vi "isUpperLevelClosed.vi"(8 "error in (no error)":errorcluster, 9 "open nodes":refnum<class "xmlNode.lvclass">[](array[class]), 10 "open names":string[](array[string]), 11 "name to close":string) -> (0 "error out":errorcluster, 1 "open nodes out":refnum<class "xmlNode.lvclass">[](array[class]), 2 "open names out":string[](array[string]))   [LabVIEW 2011, in "Tools.lvlib" / "xml.lvlib" / "XmlParser.lvclass"]
uses:
  XmlParser.lvclass
  xmlNode/xmlNode.lvclass
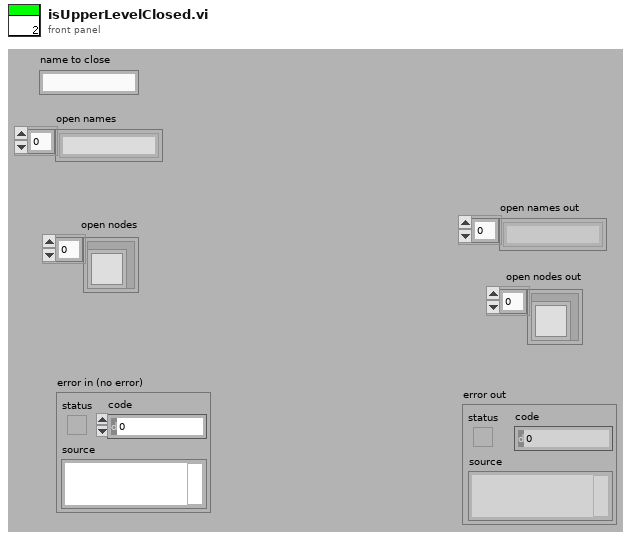
[diagram p1: front panel]
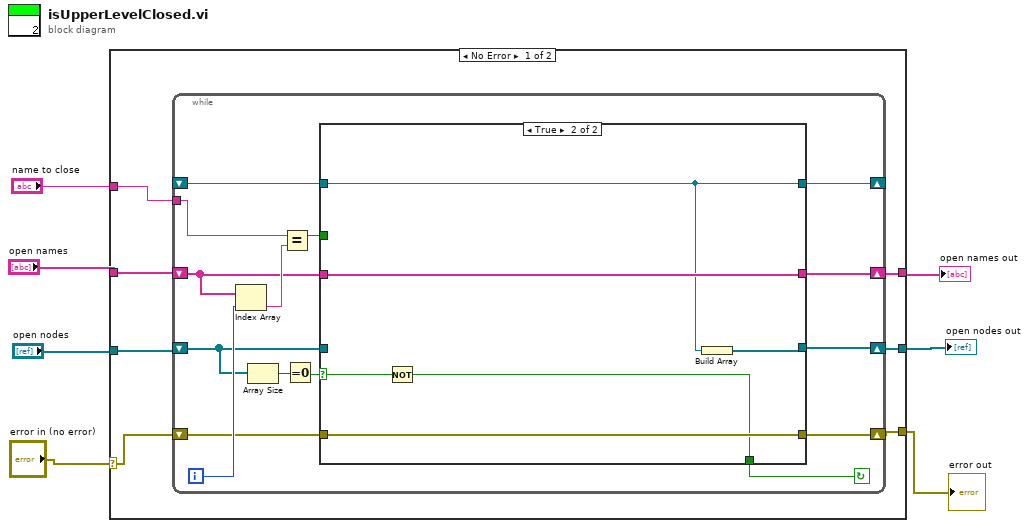
[diagram p0: block diagram]
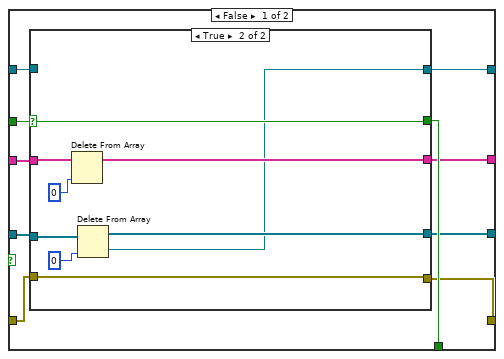
[diagram p2: hidden frame]
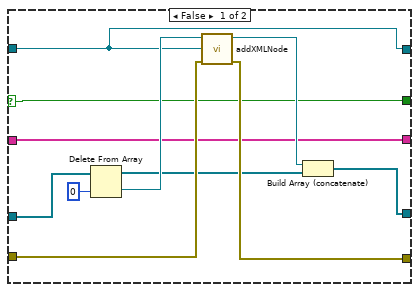
[diagram p3: hidden frame]
diagram:
  n1 = case shown="No Error" "error in (no error)" {
    selector: "error in (no error)" -> [w8 w67]
    tunnel: "open nodes" -> [w13 w66]
    tunnel: "open names" -> [w11 w68]
    tunnel: "name to close" -> [w14 _]
    tunnel: [w12 w68] -> w1
    tunnel: [w10 w67] -> w3
    tunnel: [w9 w66] -> w2
    frame No Error {
      n2 = while {
        tunnel: w14 -> [w27]
        shift-right: [w24] -> w9
        shift-left: w13 -> [w17]
        shift-right: [w23] -> w12
        shift-left: w11 -> [w22]
        shift-right: [w21] -> _
        shift-left: _ -> [w20]
        shift-right: [w19] -> w10
        shift-left: w8 -> [w18]
        i -> [w28]
        stop <- w25 continue-if-true
        n3 = Index Array(array=w22, index=w28) -> (element=w29:string)
        n4 = Array Size(array=w17) -> (size(s)=w16:i32)
        n5 = Equal?(x=w27, y=w29) -> (x = y?=w26:bool)
        n6 = Equal To 0?(x=w16) -> (x = 0?=w15:bool)
        n7 = case shown="True" w15 {
          selector: w15 -> [_ w64]
          tunnel: w26 -> [w39 _]
          tunnel: [w38 w62] -> w25
          tunnel: [w37 w61] -> w24
          tunnel: [w36 w65] -> w23
          tunnel: w22 -> [w35 w65]
          tunnel: [w34 w60] -> w21
          tunnel: w20 -> [w33 w60]
          tunnel: [w32 w63] -> w19
          tunnel: w18 -> [w31 w63]
          tunnel: w17 -> [w30 _]
          frame False {
            n8 = case shown="True" w39 {
              selector: w39 -> [w41 w59]
              tunnel: w35 -> [w40 w55]
              tunnel: w31 -> [w47 w51]
              tunnel: [w41 w59] -> w38
              tunnel: w30 -> [w50 w58]
              tunnel: [w43 w56] -> w37
              tunnel: [w40 w53] -> w36
              tunnel: [w42 w52] -> w34
              tunnel: w33 -> [w42 _]
              tunnel: [w46 w51] -> w32
              frame False {
                n9 = Delete From Array(array=w50, index=0) -> (deleted portion=w48:refnum<class "xmlNode.lvclass">, array with subset deleted=w44:refnum<class "xmlNode.lvclass">[])  [unwired: 1 in]
                n10 = call-dynamic "addXMLNode.vi"("error in (no error)"=w47, "LabVIEW Object"=w42, "xmlNode in"=w48) -> ("error out"=w46:errorcluster, "xmlNode out"=w45:refnum<class "xmlNode.lvclass">)  [unwired: 7 in]
                n11 = Build Array (concatenate)(w45, w44) -> (w43:refnum<class "xmlNode.lvclass">[])
              }
              frame True {
                n12 = Delete From Array(array=w55, index=0) -> (array with subset deleted=w53:string[])  [unwired: 1 in, 1 out]
                n13 = Delete From Array(array=w58, index=0) -> (deleted portion=w52:refnum<class "xmlNode.lvclass">, array with subset deleted=w56:refnum<class "xmlNode.lvclass">[])  [unwired: 1 in]
              }
            }
          }
          frame True {
            n14 = Not(x=w64) -> (.not. x?=w62:bool)
            n15 = Build Array(w60) -> (w61:refnum<class "xmlNode.lvclass">[])
          }
        }
      }
    }
    frame Error {
    }
  }
  "error out" <- w3
  "open nodes out" <- w2
  "open names out" <- w1
